vi "CloseComAndFt.vi"(0 "ComPort":refnum<visa-resource-name>, 11 "error in (no error)":errorcluster, 12 "Skip(T)":bool, 13 "KillFT(t)":bool caption="KillFt(t)") -> (3 "FieldTestOpen?(t)":bool, 15 "error out":errorcluster)   [LabVIEW 2018]
panel:
  out "number of replacements 2":i32
  out "FtSvcOpen?(t)":bool
  out "standard output":string
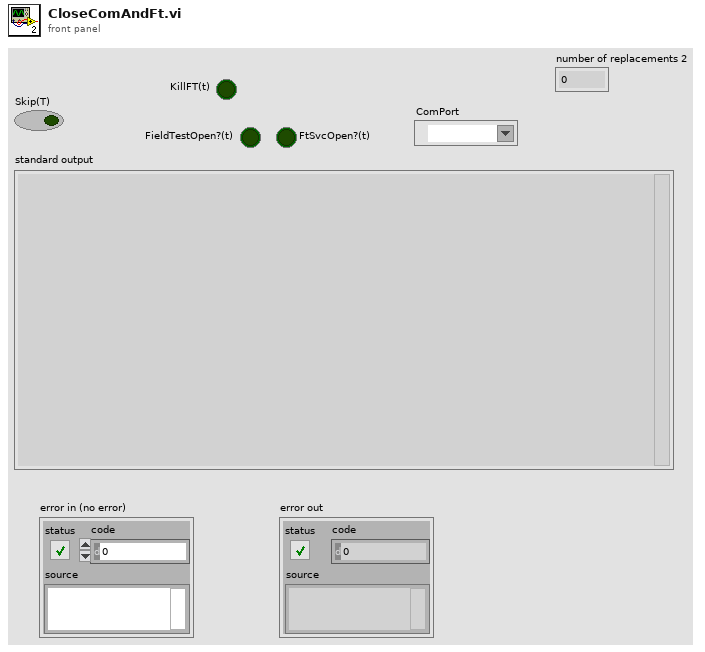
[diagram p1: front panel]
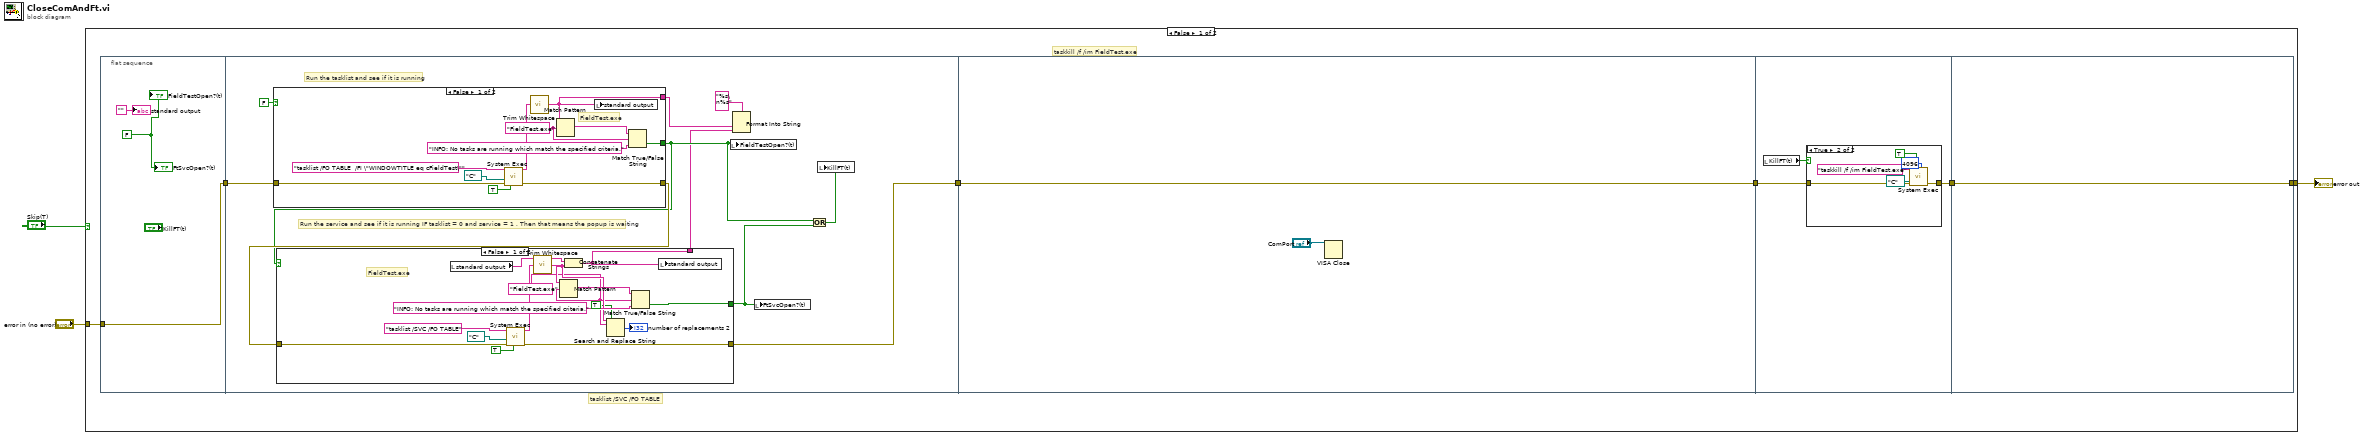
[diagram p0: block diagram]
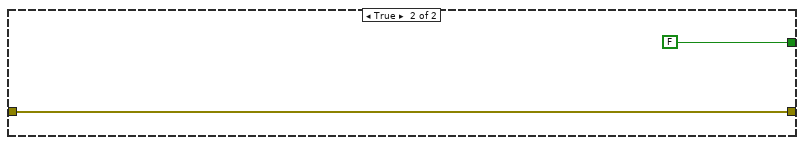
[diagram p2: hidden frame]
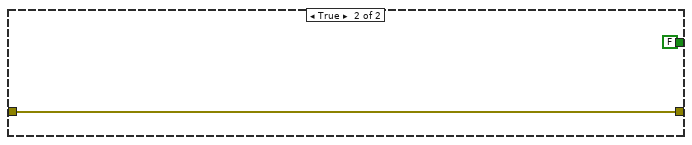
[diagram p3: hidden frame]
diagram:
  n1 = case shown="False" "Skip(T)" {
    tunnel: [w6 w66] -> w3
    tunnel: "error in (no error)" -> [w5 w66]
    frame False {
      # "tasklist /SVC /FO TABLE"
      # "taskkill /f /im FieldTest.exe"
      n2 = flat-sequence {
        tunnel: [w11] -> w9
        tunnel: w5 -> [w11]
        tunnel: w9 -> [w22]
        tunnel: [w20] -> w8
        tunnel: w8 -> [w54]
        tunnel: [w54] -> w4
        tunnel: [w56] -> w7
        tunnel: w4 -> [w57]
        tunnel: [w65] -> w6
        tunnel: w7 -> [w65]
        frame #0 {
          w10 = FALSE ("OpenNewFT(t)")
          "standard output" <- ""
          "FieldTestOpen?(t)" <- w10
          "FtSvcOpen?(t)" <- w10
        }
        frame #1 {
          # "Run the service and see if it is running IF tasklist = 0 and service = 1 , Then that means the popup is waiting"
          # "Run the tasklist and see if it is running"
          n3 = case shown="False" FALSE {
            tunnel: [w46 FALSE ("selection")] -> w18
            tunnel: w22 -> [w42 w52]
            tunnel: [w41 w52] -> w21
            tunnel: [w40 _] -> w15
            frame False {
              w44 = "FieldTest.exe" ("string")
              # "FieldTest.exe"
              n4 = call <vilib>:"System Exec.vi"("run minimized? (F)"=TRUE, "error in (no error)"=w42, "working directory"=path "C:/", "command line"="tasklist /FO TABLE  /FI \"WINDOWTITLE eq cFieldTest\"") -> ("error out"=w41:errorcluster, "standard output"=w49:string)  [unwired: 4 in, 2 out]
              n5 = call <vilib>:"Trim Whitespace.vi"("string"=w49) -> ("trimmed string"=w40:string)  [unwired: 1 in]
              n6 = Match Pattern(string=w40, regular expression=w44) -> (match substring=w43:string)  [unwired: 1 in, 3 out]
              n7 = local write "standard output"(w40) -> ()
              n8 = Match True/False String(2:"INFO: No tasks are running which match the specified criteria." ("false string"), 3:w44, 4:w43) -> (0:w46:bool)  [unwired: 1 out]
            }
            frame True {
            }
          }
          n9 = case shown="False" w18 {
            tunnel: [w33 FALSE ("selection")] -> w17
            tunnel: w21 -> [w30 w39]
            tunnel: [w29 w39] -> w20
            tunnel: [w23 _] -> w13
            frame False {
              w25 = "FieldTest.exe" ("string")
              # "FieldTest.exe"
              n10 = local read "standard output"() -> (w28:string)
              n11 = call <vilib>:"System Exec.vi"("run minimized? (F)"=TRUE, "error in (no error)"=w30, "working directory"=path "C:/", "command line"="tasklist /SVC /FO TABLE") -> ("error out"=w29:errorcluster, "standard output"=w36:string)  [unwired: 4 in, 2 out]
              n12 = call <vilib>:"Trim Whitespace.vi"("string"=w36) -> ("trimmed string"=w27:string)  [unwired: 1 in]
              n13 = Match Pattern(string=w27, regular expression=w25) -> (match substring=w31:string)  [unwired: 1 in, 3 out]
              n14 = Concatenate Strings(w28, w27) -> (w23:string)
              n15 = Search and Replace String(replace all?=TRUE ("replace all? (F)"), input string=w27, search string=w25) -> (number of replacements=→"number of replacements 2":i32)  [unwired: 5 in, 3 out]
              n16 = Match True/False String(2:"INFO: No tasks are running which match the specified criteria." ("false string"), 3:w25, 4:w31) -> (0:w33:bool)  [unwired: 1 out]
              n17 = local write "standard output"(w23) -> ()
            }
            frame True {
            }
          }
          n18 = local write "FieldTestOpen?(t)"(w18) -> ()
          n19 = Format Into String(format string="%s\n%s", w15, w13) -> ()  [unwired: 2 in, 2 out]
          n20 = local write "FtSvcOpen?(t)"(w17) -> ()
          n21 = Or(x=w18, y=w17) -> (x .or. y?=w16:bool)
          n22 = local write "KillFT(t)"(w16) -> ()
        }
        frame #2 {
          n23 = VISA Close(VISA resource name="ComPort") -> ()  [unwired: 1 in, 1 out]
        }
        frame #3 {
          n24 = local read "KillFT(t)"() -> (w55:bool)
          n25 = case shown="True" w55 {
            tunnel: w57 -> [w58 w63]
            tunnel: [w58 w62] -> w56
            frame False {
            }
            frame True {
              n26 = call <vilib>:"System Exec.vi"("expected output size  (4096)"=u32 4096, "wait until completion? (T)"=TRUE, "error in (no error)"=w63, "working directory"=path "C:/", "command line"="taskkill /f /im FieldTest.exe") -> ("error out"=w62:errorcluster)  [unwired: 3 in, 3 out]
            }
          }
        }
        frame #4 {
        }
      }
    }
    frame True {
    }
  }
  "error out" <- w3
